vi "osc3, multiples muestras.vi"() -> ()   [LabVIEW 2016]
uses:
  <instrlib>/Tektronix TDS 200 1000 2000 Series/Public/Data/Read (Single Waveform).vi
  <instrlib>/Tektronix TDS 200 1000 2000 Series/Tektronix TDS 200 1000 2000 Series.lvlib
panel:
  out "Measurement":dbl
  in  "Stop Button":bool
  in  "VISA resource name":refnum<visa-resource-name>
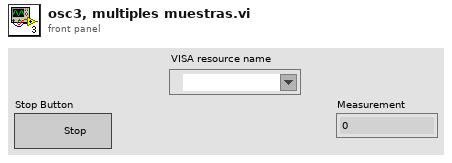
[diagram p1: front panel]
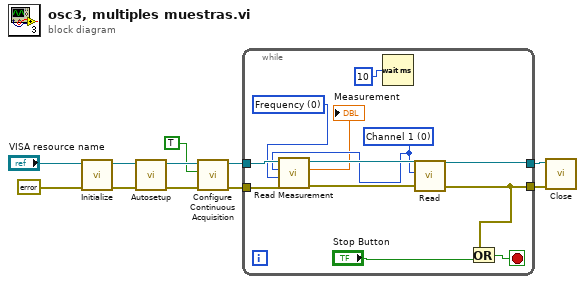
[diagram p0: block diagram]
diagram:
  n1 = call <instrlib>:"Initialize.vi"("error in (no error)"=errorcluster {"status"=FALSE, "code"=0, "source"=""}, "VISA resource name"="VISA resource name") -> ("error out"=w10:errorcluster, "VISA resource name out"=w11:refnum<visa-resource-name>)  [unwired: 8 in]
  n2 = call <instrlib>:"Autosetup.vi"("error in (no error)"=w10, "VISA resource name"=w11) -> ("error out"=w7:errorcluster, "VISA resource name out"=w6:refnum<visa-resource-name>)  [unwired: 8 in]
  n3 = call <instrlib>:"Configure Continuous Acquisition.vi"("error in (no error)"=w7, "Enable Continuous Acquisition Mode (True)"=TRUE, "VISA resource name"=w6) -> ("error out"=w4:errorcluster, "VISA resource name out"=w3:refnum<visa-resource-name>)  [unwired: 7 in]
  n4 = while {
    tunnel: w4 -> [w17]
    tunnel: w3 -> [w18]
    tunnel: [w22] -> w2
    tunnel: [w21] -> w1
    stop <- w19 stop-if-true
    w14 = 0 items=["Frequency", "Mean", "Period", "Pulse Duty", "Peak to Peak", "Cycle RMS", "Minimum", "Maximum", "Rise Time", "Fall Time", "Positive Width", "Negative Width", "Amplitude", "Cycle Mean", "High", "Low", "Negative Duty", "Positive Overshoot", "Negative Overshoot", "Cursor Mean", "Burst Width", "Positive Pulse Count", "Negative Pulse Count", "Rising Edge Count", "Falling Edge Count", "Area", "Cycle Area", "RMS", "Cursor RMS"] ("Measurement Type (0: Frequency)")
    w13 = u16 0 items=["Channel 1", "Channel 2", "Channel 3", "Channel 4", "Math", "Reference A", "Reference B", "Reference C", "Reference D", "FFT"] ("Source (0: Channel 1)")
    n5 = call <instrlib>:"Read Measurement.vi"("error in (no error)"=w17, "Measurement Type (0: Frequency)"=w14, "Channel (1: Channel 1)"=w13, "VISA resource name"=w18) -> ("error out"=w15:errorcluster, "Measurement"=→"Measurement":dbl, "VISA resource name out"=w16:refnum<visa-resource-name>)  [unwired: 4 in, 1 out]
    n6 = Wait (ms)(milliseconds to wait=u32 10) -> ()  [unwired: 1 out]
    n7 = call-poly <instrlib>:"Read.vi"("error in (no error)"=w15, "Source (0: Channel 1)"=w13, "VISA resource name"=w16) -> ("error out"=w21:errorcluster, "VISA resource name out"=w22:refnum<visa-resource-name>)  [unwired: 6 in, 1 out]
    n8 = Or(x=w21, y="Stop Button") -> (x .or. y?=w19:bool)
  }
  n9 = call <instrlib>:"Close.vi"("error in (no error)"=w1, "VISA resource name"=w2) -> ()  [unwired: 9 in, 1 out]
